vi "GetPosSingleAxis.vi"(8 "error in (no error)":errorcluster caption="entrée d'erreur (pas d'erreur)", 10 "Axis":i32=1 min=1 max=4, 11 "DelayLineLS4 en entrée":refnum<class "DelayLineLS4.lvclass">) -> (0 "error out":errorcluster caption="sortie d'erreur", 2 "Pos":dbl, 3 "DelayLineLS4 en sortie":refnum<class "DelayLineLS4.lvclass">)   [LabVIEW 2015, in "DelayLineLS4.lvclass"]
uses:
  DelayLineLS4.lvclass
  DelayLine.lvclass/DelayLine.ctl
  <vilib>/Utility/error.llb/DialogType.ctl
  <vilib>/ErrorRing/Error Ring.xnode
  DelayLine.lvclass
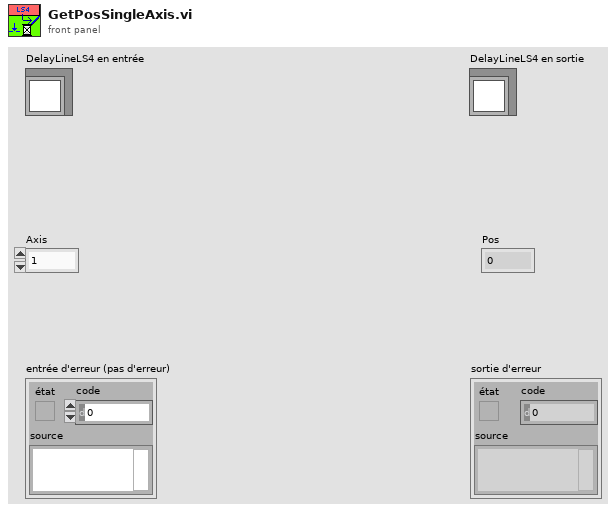
[diagram p1: front panel]
types:
  T1 = typedef "DialogType.ctl" = u16
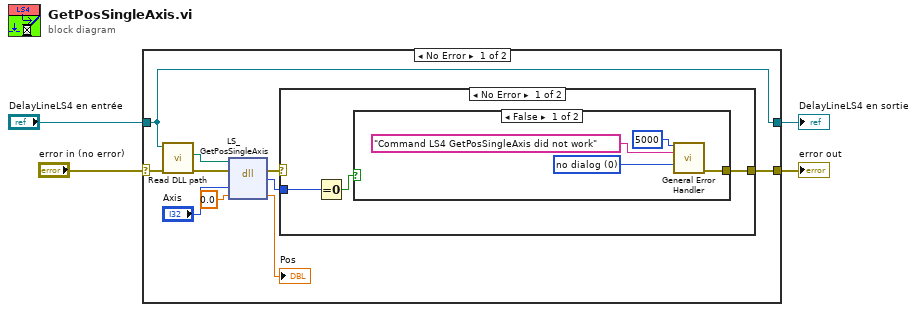
[diagram p0: block diagram]
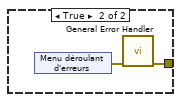
[diagram p2: hidden frame]
diagram:
  n1 = case shown="No Error" "error in (no error)" {
    selector: "error in (no error)" -> [w13 w27]
    tunnel: [w8 w27] -> w3
    tunnel: [w14 w26] -> w1
    tunnel: "DelayLineLS4 en entrée" -> [w14 w26]
    frame No Error {
      n2 = call "Read DLL path.vi"("error in (no error)"=w13, "DelayLine in"=w14) -> ("error out"=w10:errorcluster, "DLL path"=w11:path)  [unwired: 7 in, 1 out]
      n3 = dll-call lib="G:/SD/TRANCON/DLL/LStep4.dll" fn="LS_GetPosSingleAxis"(path in=w11, error in=w10, "Axis"="Axis", "Pos"=0.0) -> (error out=w7:errorcluster, "type de retour"=w9:i32, "Pos"=→"Pos":dbl)  [unwired: 2 in, 1 out]
      n4 = case shown="No Error" w7 {
        selector: w7 -> [_ w25]
        tunnel: w9 -> [w17 _]
        tunnel: [w15 w25] -> w8
        frame No Error {
          n5 = Equal To 0?(x=w17) -> (x = 0?=w16:bool)
          n6 = case shown="False" w16 {
            tunnel: [w19 w22] -> w15
            frame False {
              w18 = T1 0 items=["no dialog", "OK message", "continue or stop message", "OK message + warnings", "continue/stop + warnings"] ("type of dialog (OK msg:1)")
              n7 = call <vilib>:"General Error Handler.vi"("[error code] (0)"=5000 ("code"), "[error source] (\" \")"="Command LS4 GetPosSingleAxis did not work" ("String to Prepend to source (\"\")"), "type of dialog (OK msg:1)"=w18) -> ("error out"=w19:errorcluster)  [unwired: 8 in, 4 out]
            }
            frame True {
              n8 = xnode "Menu déroulant d'erreurs"() -> ("error out"=w23:errorcluster)
              n9 = call <vilib>:"General Error Handler.vi"("error in (no error)"=w23) -> ("error out"=w22:errorcluster)  [unwired: 10 in, 4 out]
            }
          }
        }
        frame Error {
        }
      }
    }
    frame Error {
    }
  }
  "error out" <- w3
  "DelayLineLS4 en sortie" <- w1
